vi "J-KEM_subVI_no_control.vi"(10 "Address in":T1, 11 "J-KEM on?":bool) -> (0 "Temp (C)":dbl format="%#_6f", 1 "String data out":string, 2 "plot data out":cluster{"Numeric Control":dbl} {"Numeric Control" format="%#_6f"}, 3 "Address out":T1)   [LabVIEW 2014]
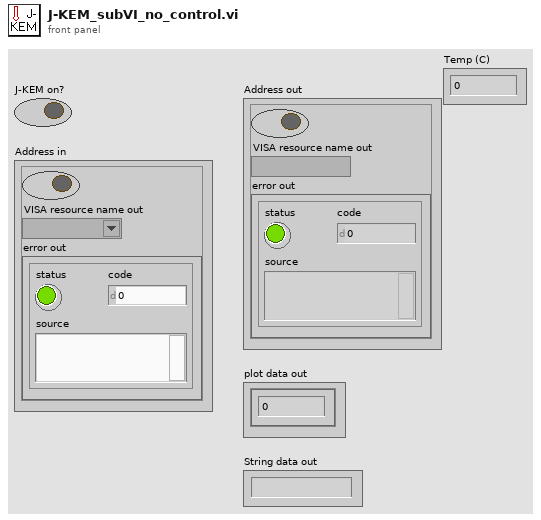
[diagram p1: front panel]
types:
  T1 = cluster{"Boolean":bool, "VISA resource name out":refnum<visa-resource-name>, "error out":errorcluster}
  T2 = cluster{bool, "VISA resource name out":refnum<visa-resource-name>, "error out":errorcluster}
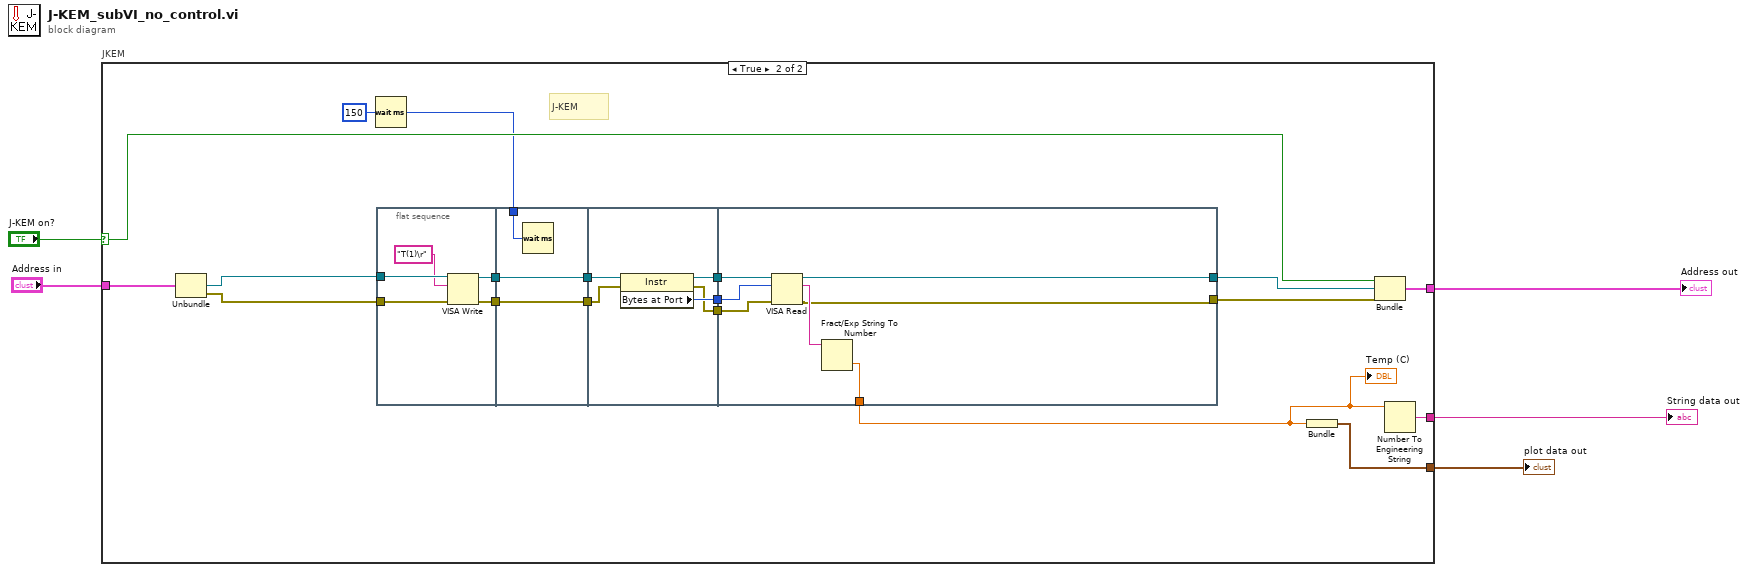
[diagram p0: block diagram]
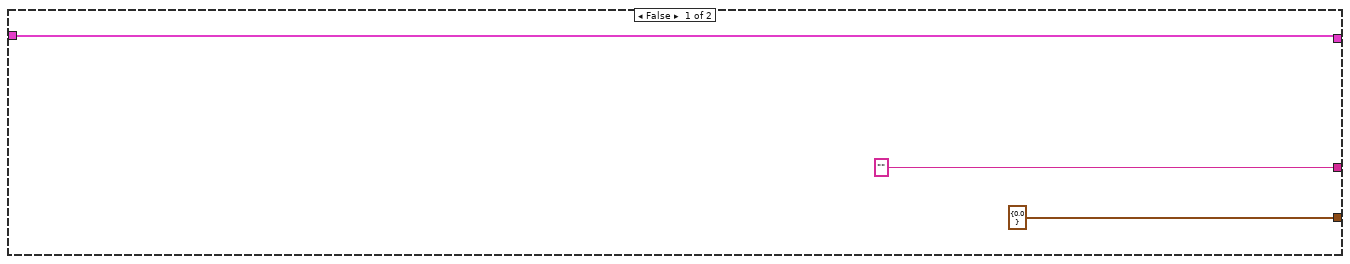
[diagram p2: hidden frame]
diagram:
  n1 = case "JKEM" shown="True" "J-KEM on?" {
    selector: "J-KEM on?" -> [_ w20]
    tunnel: "Address in" -> [w8 w24]
    tunnel: [w8 w22] -> w2
    tunnel: ["" w21] -> w3
    tunnel: [cluster{dbl} {0.0} w18] -> w5
    frame False {
    }
    frame True {
      w9 = u32 150 ("milliseconds to wait")
      # "J-KEM"
      n2 = Unbundle(w24) -> ("VISA resource name out"=w23:refnum<visa-resource-name>, "error out"=w19:errorcluster)  [unwired: 1 out]
      n3 = Wait (ms)(milliseconds to wait=w9) -> ()  [unwired: 1 out]
      n4 = flat-sequence {
        tunnel: w23 -> [w31]
        tunnel: w19 -> [w30]
        tunnel: [w28] -> w16
        tunnel: [w27] -> w15
        tunnel: w9 -> [w34]
        tunnel: [w33] -> w14
        tunnel: w16 -> [w33]
        tunnel: w15 -> [w32]
        tunnel: [w32] -> w13
        tunnel: w14 -> [w39]
        tunnel: w13 -> [w38]
        tunnel: [w37] -> w12
        tunnel: [w36] -> w11
        tunnel: [w35] -> w10
        tunnel: [w46] -> w25
        tunnel: [w40] -> w26
        tunnel: [w41] -> w17
        tunnel: w10 -> [w43]
        tunnel: w11 -> [w44]
        tunnel: w12 -> [w45]
        frame #0 {
          n5 = VISA Write(VISA resource name=w31, write buffer="T(1)\r", error in (no error)=w30) -> (VISA resource name out=w28:refnum<visa-resource-name>, error out=w27:errorcluster)  [unwired: 1 out]
        }
        frame #1 {
          n6 = Wait (ms)(milliseconds to wait=w34) -> ()  [unwired: 1 out]
        }
        frame #2 {
          n7 = property class="Instr"(reference=w39, error in=w38) -> (reference out=w37:refnum<visa-resource-name>, error out=w35:errorcluster, "Bytes at Port"=w36:u32)
        }
        frame #3 {
          n8 = VISA Read(VISA resource name=w45, byte count=w44, error in (no error)=w43) -> (VISA resource name out=w46:refnum<visa-resource-name>, read buffer=w42:string, error out=w40:errorcluster)  [unwired: 1 out]
          n9 = Fract/Exp String To Number(string=w42) -> (number=w41:dbl)  [unwired: 3 in, 1 out]
        }
      }
      n10 = Bundle(w17) -> (w18:cluster{dbl})  [unwired: 1 in]
      n11 = Bundle(w20, "VISA resource name out"=w25, "error out"=w26) -> (w22:T2)  [unwired: 1 in]
      n12 = Number To Engineering String(4:w17) -> (0:w21:string)  [unwired: 3 in]
      "Temp (C)" <- w17
    }
  }
  "plot data out" <- w5
  "String data out" <- w3
  "Address out" <- w2
